vi "EnqueuebyName.vi"(6 "Loop Name":string, 7 "Instance":i32, 8 "error in (no error)":errorcluster, 10 "Data":variant, 11 "Msg":string) -> (0 "error out":errorcluster)   [LabVIEW 2017, in "Communication.lvlib"]
uses:
  Communication.lvlib
  SubVIs/MsgData.ctl
  SubVIs/MsgAck.ctl
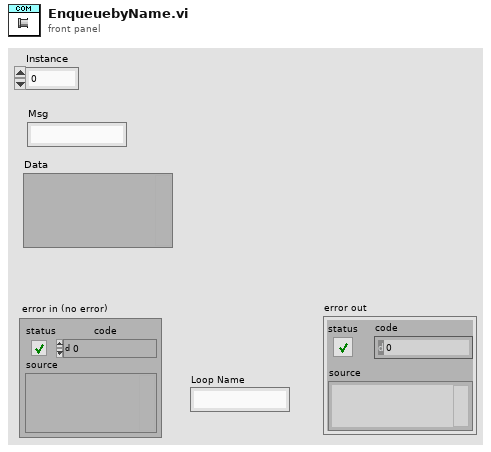
[diagram p1: front panel]
types:
  T1 = typedef "Communication.lvlib/MsgData.ctl" = cluster{"Msg":string, "Data":variant, "Ack":refnum<notifier>}
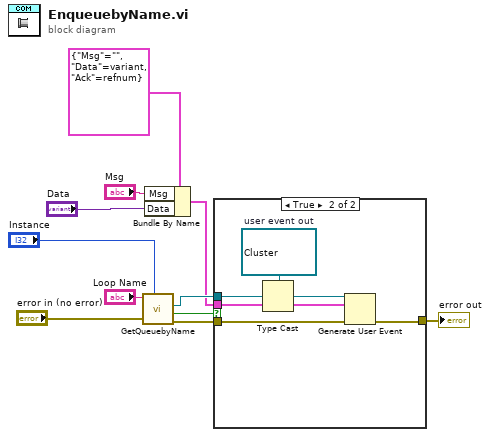
[diagram p0: block diagram]
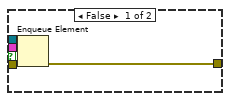
[diagram p2: hidden frame]
diagram:
  n1 = call "GetQueuebyName.vi"("Instance"="Instance", "error in (no error)"="error in (no error)", "Name"="Loop Name") -> ("error out"=w9:errorcluster, "Event?"=w2:bool, "queue out"=w8:refnum<queue>)  [unwired: 6 in]
  n2 = Bundle By Name(cluster=T1 {"Msg"="", "Data"=variant, "Ack"=refnum} ("element"), "Msg"="Msg", "Data"="Data") -> (w6:T1)
  n3 = case shown="True" w2 {
    tunnel: w9 -> [w15 w19]
    tunnel: w8 -> [w14 w21]
    tunnel: w6 -> [w13 w17]
    tunnel: [w12 w16] -> w3
    frame False {
      n4 = Enqueue Element(queue=w14, element=w13, error in (no error)=w15) -> (error out=w12:errorcluster)  [unwired: 1 in, 2 out]
    }
    frame True {
      w20 = refnum<user-event> refnum  # user event out
      n5 = Type Cast(type=w20, x=w21) -> (*(type *) &x=w18:refnum<user-event>)
      n6 = Generate User Event(user event=w18, event data cluster=w17, error in=w19) -> (error out=w16:errorcluster)  [unwired: 1 in, 1 out]
    }
  }
  "error out" <- w3
